vi "CameraConnect.vi"(8 "error in (no error)":errorcluster, 9 "serial":u64 format="%x", 10 "name":string, 11 "AndorSDK3 in":refnum<class "Andor3.lvclass">) -> (0 "error out":errorcluster, 2 "CameraInfo":T1 {"serial" format="%x"}, 3 "AndorSDK3 out":refnum<class "Andor3.lvclass">)   [LabVIEW 2010, in "Andor3.lvclass"]
uses:
  <userlib>/bias2/classes/Andor3/Andor3.lvclass
  <userlib>/bias2/classes/CameraBase/CameraInfo.ctl
  <userlib>/bias2/classes/Andor3/Andor3.lvclass/Andor3.ctl
  <userlib>/bias2/classes/CameraBase/CameraBase.lvclass
  <userlib>/atcoreA/atcoreA.lvlib
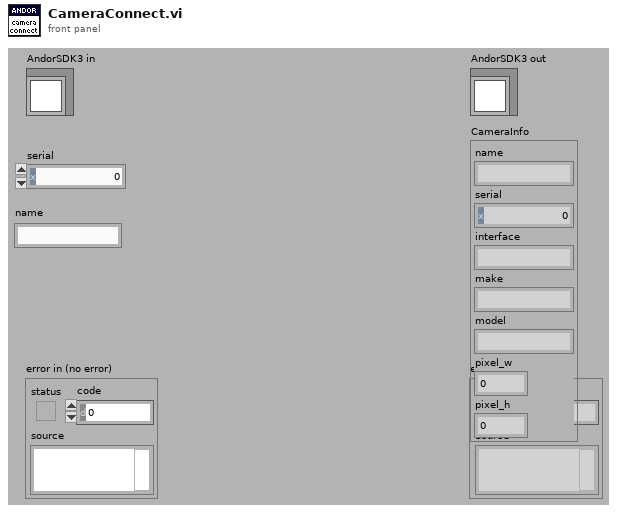
[diagram p1: front panel]
types:
  T1 = typedef "CameraInfo.ctl" = cluster{"name":string, "serial":u64, "interface":string, "make":string, "model":string, "pixel_w":dbl, "pixel_h":dbl}
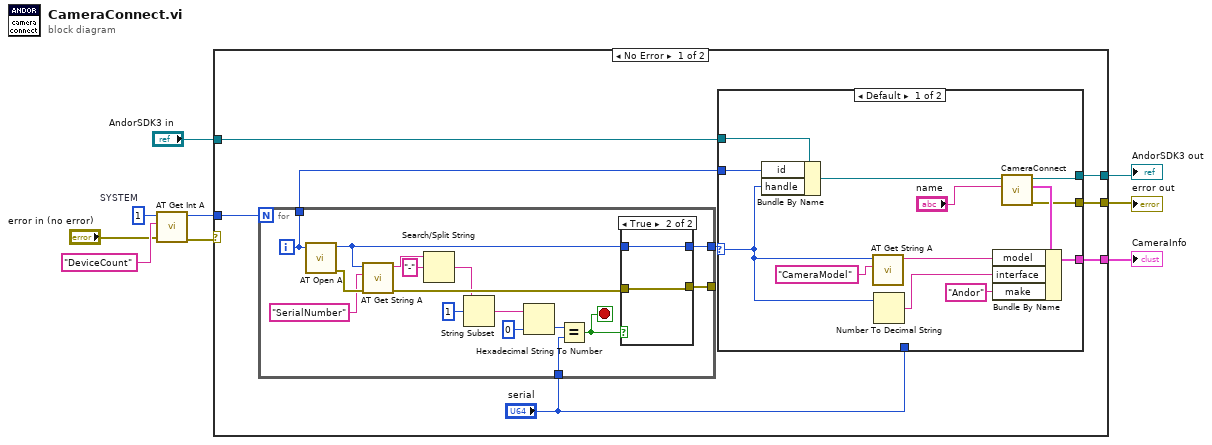
[diagram p0: block diagram]
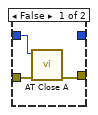
[diagram p2: hidden frame]
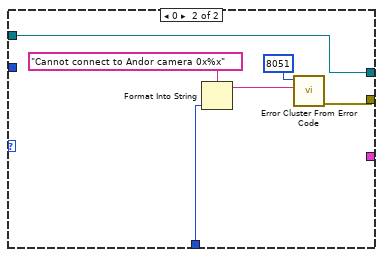
[diagram p3: hidden frame]
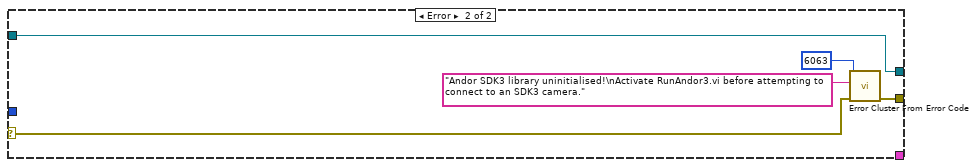
[diagram p4: hidden frame]
diagram:
  w4 = 1  # SYSTEM
  n1 = call <userlib>:"AT Get Int A.vi"("error in (no error)"="error in (no error)", "Feature"="DeviceCount", "Hndl"=w4) -> ("error out"=w2:errorcluster, "Value"=w5:i64)  [unwired: 7 in]
  n2 = case shown="No Error" w2 {
    selector: w2 -> [_ w59]
    tunnel: [w17 w58] -> w9
    tunnel: [w16 _] -> w8
    tunnel: [w15 w62] -> w7
    tunnel: w5 -> [w14 _]
    tunnel: "AndorSDK3 in" -> [w10 w58]
    frame No Error {
      n3 = for {
        N: w14 -> [_]
        tunnel: "serial" -> [w30]
        tunnel: [w26] -> w13
        tunnel: [w25] -> w12
        tunnel: [w24] -> _
        i -> [w25]
        stop <- w27 stop-if-true
        n4 = call <userlib>:"AT Open A.vi"("CameraIndex"=w25) -> ("error out"=w33:errorcluster, "Hndl"=w29:i32)  [unwired: 9 in]
        n5 = call <userlib>:"AT Get String A.vi"("error in (no error)"=w33, "Feature"="SerialNumber", "Hndl"=w29) -> ("error out"=w28:errorcluster, "String"=w21:string)  [unwired: 7 in]
        n6 = Search/Split String(string=w21, search string/char (-)="-") -> (match + rest of string=w20:string)  [unwired: 1 in, 2 out]
        n7 = String Subset(string=w20, offset (0)=1) -> (substring=w22:string)  [unwired: 1 in]
        n8 = Hexadecimal String To Number(string=w22, default (0uL)=u64 0 ("default (0 U32)")) -> (number=w31:u64)  [unwired: 1 in, 1 out]
        n9 = Equal?(x=w31, y=w30) -> (x = y?=w27:bool)
        n10 = case shown="True" w27 {
          tunnel: w29 -> [w36 w37]
          tunnel: [w35 w38] -> w24
          tunnel: w28 -> [w34 w38]
          tunnel: [_ w37] -> w26
          frame False {
            n11 = call <userlib>:"AT Close A.vi"("error in (no error)"=w34, "Hndl"=w36) -> ("error out"=w35:errorcluster)  [unwired: 9 in]
          }
          frame True {
          }
        }
      }
      n12 = case shown="Default" w13 {
        selector: w13 -> [w41 _]
        tunnel: w10 -> [w51 w57]
        tunnel: [w47 w57] -> w17
        tunnel: [w48 _] -> w16
        tunnel: [w43 w53] -> w15
        tunnel: w12 -> [w42 _]
        tunnel: "serial" -> [_ w52]
        frame Default {
          n13 = Bundle By Name(cluster=w51, "id"=w42, "handle"=w41) -> (w46:refnum<class "Andor3.lvclass">)
          n14 = call <userlib>:"AT Get String A.vi"("Feature"="CameraModel", "Hndl"=w41) -> ("String"=w39:string)  [unwired: 8 in, 1 out]
          n15 = Number To Decimal String(number=w41) -> (decimal integer string=w45:string)  [unwired: 1 in]
          n16 = call-parent "CameraConnect.vi"("name"="name", "CameraBase in"=w46) -> ("error out"=w43:errorcluster, "CameraInfo"=w49:T1, "CameraBase out"=w47:refnum<class "Andor3.lvclass">)  [unwired: 7 in]
          n17 = Bundle By Name(cluster=w49, "model"=w39, "interface"=w45, "make"="Andor") -> (w48:T1)
        }
        frame 0 {
          n18 = Format Into String(format string="Cannot connect to Andor camera 0x%x", w52) -> (resulting string=w55:string)  [unwired: 2 in, 1 out]
          n19 = call <vilib>:"Error Cluster From Error Code.vi"("error message (\"\")"=w55, "error code (0)"=8051) -> ("error out"=w53:errorcluster)  [unwired: 7 in]
        }
      }
    }
    frame Error {
      n20 = call <vilib>:"Error Cluster From Error Code.vi"("error in (no error)"=w59, "error message (\"\")"="Andor SDK3 library uninitialised!\nActivate RunAndor3.vi before attempting to connect to an SDK3 camera." ("error message (\"\")"), "error code (0)"=6063) -> ("error out"=w62:errorcluster)  [unwired: 6 in]
    }
  }
  "error out" <- w7
  "AndorSDK3 out" <- w9
  "CameraInfo" <- w8
